vi "Day 1 (Part Two).vi"() -> ()   [LabVIEW 2021]
uses:
  7385093b-823c-42d4-ac89-861aca289567.vi
  <vilib>/Comparison/Less/Less Functor/Less Functor.lvclass
panel:
  out "Top Three Sum":u32
  out "Unique Sum?":bool
  out "Maximum Value":u32
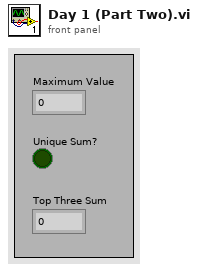
[diagram p1: front panel]
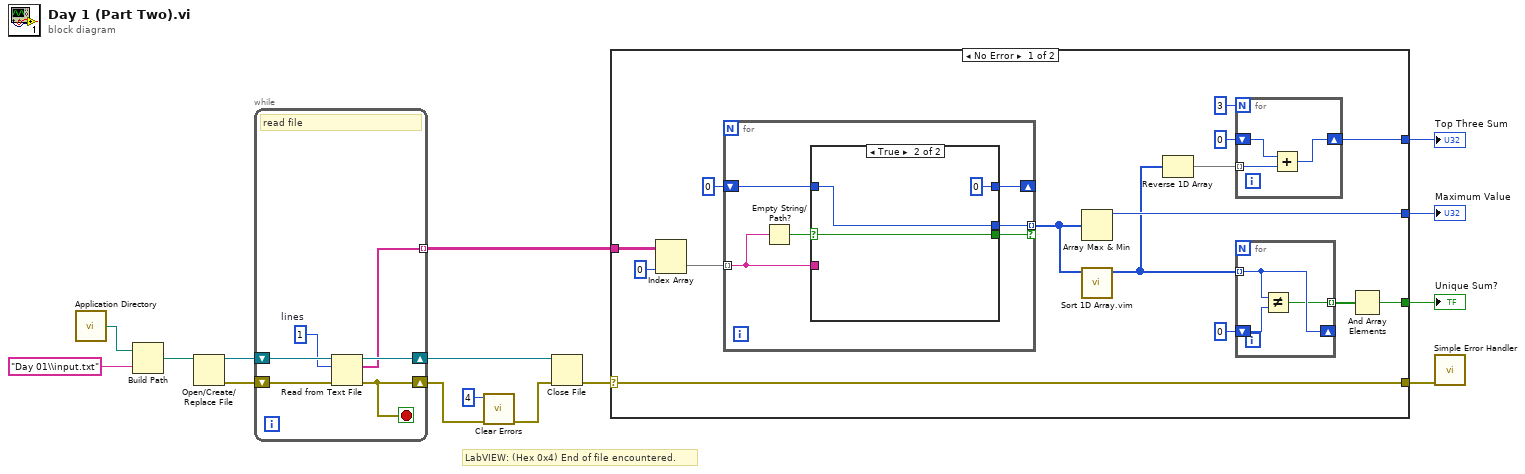
[diagram p0: block diagram]
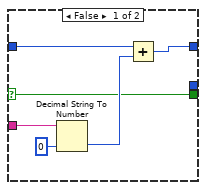
[diagram p2: hidden frame]
diagram:
  # "LabVIEW: (Hex 0x4) End of file encountered."
  n1 = call <vilib>:"Application Directory.vi"() -> ("Application Directory"=w15:path)
  n2 = Build Path(base path=w15, name or relative path="Day 01\\input.txt") -> (appended path=w13:path)
  n3 = Open/Create/Replace File(file path (use dialog)=w13) -> (refnum out=w11:refnum<file>, error out=w12:errorcluster)  [unwired: 5 in, 1 out]
  n4 = while {
    shift-right: [w16] -> w9
    shift-left: w12 -> [w21]
    shift-right: [w19] -> w10
    shift-left: w11 -> [w20]
    tunnel: [w17] -> w6 mode=indexing
    stop <- w16 stop-if-true
    w18 = 1  # lines
    # "read file"
    n5 = Read from Text File(file (use dialog)=w20, count=w18, error in=w21) -> (refnum out=w19:refnum<file>, text=w17:string[], error out=w16:errorcluster)  [unwired: 1 in, 1 out]
  }
  n6 = call <vilib>:"Clear Errors.vi"("error in (no error)"=w9, "specific error code to clear (0: all)"=4) -> ("error out"=w7:errorcluster)  [unwired: 4 in, 1 out]
  n7 = Close File(refnum=w10, error in=w7) -> (error out=w5:errorcluster)  [unwired: 1 out]
  n8 = case shown="No Error" w5 {
    selector: w5 -> [w27 w58]
    tunnel: w6 -> [w36 _]
    tunnel: [w29 _] -> w4
    tunnel: [w28 _] -> w3
    tunnel: [w27 w58] -> w2
    tunnel: [w22 _] -> w1
    frame No Error {
      n9 = Index Array(array=w36, index (col)=0 ("disabled index (col)")) -> (element=w34:string[])  [unwired: 1 in]
      n10 = for {
        tunnel: w34 -> [w47] mode=indexing
        shift-right: [w45] -> _
        shift-left: u32 0 -> [w46]
        tunnel: [w44] -> w32 mode=indexing if=w43
        n11 = Empty String/Path?(string/path=w47) -> (empty?=w48:bool)
        n12 = case shown="True" w48 {
          selector: w48 -> [w49 w55]
          tunnel: w47 -> [w54 _]
          tunnel: w46 -> [w51 w56]
          tunnel: [w50 u32 0] -> w45
          tunnel: [_ w56] -> w44
          tunnel: [w49 w55] -> w43
          frame False {
            n13 = Decimal String To Number(string=w54, default (0L)=u32 0 ("default (0 I32)")) -> (number=w52:u32)  [unwired: 1 in, 1 out]
            n14 = Add(x=w51, y=w52) -> (x+y=w50:u32)
          }
          frame True {
          }
        }
      }
      n15 = Array Max & Min(array=w32) -> (max value=w29:u32)  [unwired: 3 out]
      n16 = call "Sort 1D Array.vim"("unsorted array"=w32) -> ("sorted array"=w26:u32[])  [unwired: 10 in]
      n17 = Reverse 1D Array(array=w26) -> (reversed array=w25:u32[])
      n18 = for {
        N: 3 -> [_]
        tunnel: w25 -> [w39] mode=indexing
        shift-right: [w38] -> w22
        shift-left: u32 0 -> [w37]
        n19 = Add(x=w37, y=w39) -> (x+y=w38:u32)
      }
      n20 = for {
        tunnel: w26 -> [w42] mode=indexing
        shift-right: [w42] -> _
        shift-left: u32 0 -> [w41]
        tunnel: [w40] -> w30 mode=indexing
        n21 = Not Equal?(x=w42, y=w41) -> (x != y?=w40:bool)
      }
      n22 = And Array Elements(Boolean array=w30) -> (logical AND=w28:bool)
    }
    frame Error {
    }
  }
  "Maximum Value" <- w4
  "Unique Sum?" <- w3
  "Top Three Sum" <- w1
  n23 = call <vilib>:"Simple Error Handler.vi"("error in (no error)"=w2) -> ()  [unwired: 4 in, 5 out]
